vi "DaqOpen.vi"(8 "error in":errorcluster caption="错误输入", 10 "扫描速率[S/s]":dbl=25000.0 min=0.0 format="%.2f", 11 "通道输入":tag="cDAQ2Mod1/ai0") -> (0 "error out":errorcluster caption="错误输出", 3 "task out":refnum<k21> caption="任务输出")   [LabVIEW 2020]
uses:
  <vilib>/DAQmx/create/channels.llb/DAQmx Create Channel (AI-Voltage-Basic).vi
  <vilib>/DAQmx/configure/timing.llb/DAQmx Timing (Sample Clock).vi
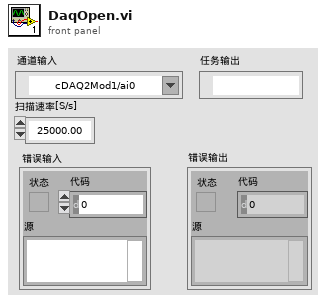
[diagram p1: front panel]
types:
  T1 = cluster{"coupling":i32, "enable excitation":bool, "excitation value":dbl}
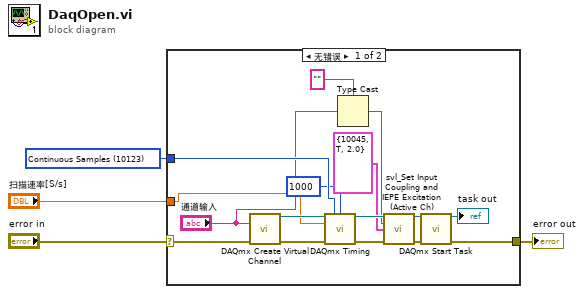
[diagram p0: block diagram]
diagram:
  w3 = 10123 items=["Finite Samples"=10178, "Continuous Samples"=10123] ("sample mode")
  n1 = case shown="无错误" "error in" {
    selector: "error in" -> [w11 w21]
    tunnel: "扫描速率[S/s]" -> [w18 _]
    tunnel: w3 -> [w17 _]
    tunnel: [w8 w21] -> w1
    frame No Error {
      n2 = call-poly <vilib>:"DAQmx Create Virtual Channel.vi"("physical channels"="通道输入", "error in"=w11) -> ("task out"=w20:refnum<k21>, "error out"=w19:errorcluster)  [unwired: 12 in]
      n3 = call-poly <vilib>:"DAQmx Timing.vi"("task/channels in"=w20, "sample mode"=w17, "samples per channel"=1000, "rate"=w18, "error in"=w19) -> ("task out"=w15:refnum<k21>, "error out"=w16:errorcluster)  [unwired: 9 in]
      n4 = Type Cast(type="", x="通道输入") -> (*(type *) &x=w13:string)
      n5 = call <vilib>:"svl_Set Input Coupling and IEPE Excitation (Active Ch).vi"("AI task name"=w15, "active channels"=w13, "DSA channel settings"=T1 {"coupling"=10045, "enable excitation"=TRUE, "excitation value"=2.0}, "error in (no error)"=w16) -> ("dup AI task name"=w10:refnum<k21>, "error out"=w9:errorcluster)  [unwired: 10 in]
      n6 = call <vilib>:"DAQmx Start Task.vi"("task/channels in"=w10, "error in"=w9) -> ("task out"=→"task out":refnum<k21>, "error out"=w8:errorcluster)  [unwired: 12 in]
    }
    frame Error {
    }
  }
  "error out" <- w1
